vi "C2_yaw.vi"(0 "setpoint":dbl, 1 "PID gains":T1={"proportional gain (Kc)"=1.0, "integral time (Ti, min)"=0.01, "derivative time (Td, min)"=0.0}, 2 "Actual Heading":dbl) -> (3 "Pwm Output":dbl)   [LabVIEW 2012]
uses:
  <vilib>/addons/control/pid/pid.llb/PID (DBL).vi
  <vilib>/addons/control/pid/NI_PID_pid.lvlib
panel:
  out "Time Response":cluster{"Actual Depth (m)":dbl, "setpoint":dbl}(graph)
  out "dt out (s)":dbl
  in  "Reinitialize? (F)":bool
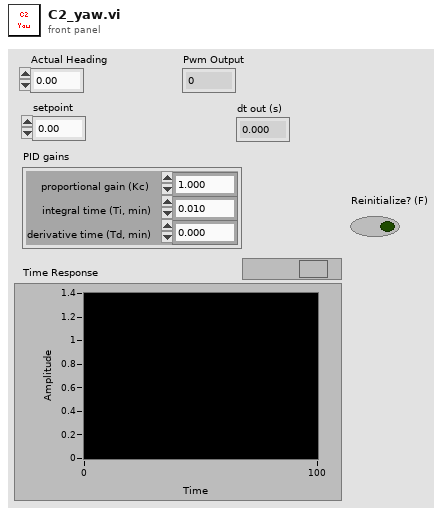
[diagram p1: front panel]
types:
  T1 = cluster{"proportional gain (Kc)":dbl, "integral time (Ti, min)":dbl, "derivative time (Td, min)":dbl}
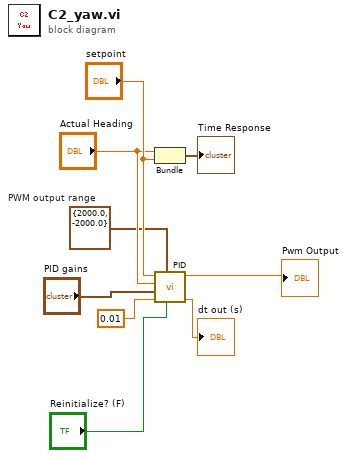
[diagram p0: block diagram]
diagram:
  w3 = cluster{"output high":dbl, "output low":dbl} {"output high"=2000.0, "output low"=-2000.0}  # PWM output range
  n1 = Bundle("Actual Heading"="Actual Heading", "setpoint"="setpoint") -> (→"Time Response":cluster{"Actual Heading":dbl, "setpoint":dbl})  [unwired: 1 in]
  n2 = call-poly <vilib>:"PID.vi"("reinitialize? (F)"="Reinitialize? (F)", "output range"=w3, "dt (s)"=0.01, "PID gains"="PID gains", "process variable"="Actual Heading", "setpoint"="setpoint") -> ("dt out (s)"=→"dt out (s)":dbl, "output"=→"Pwm Output":dbl)  [unwired: 4 in]
